vi "QuickSortinData.vi"(0 "line":u16, 2 "plane":u16, 3 "binning [ms]":dbl format="%.2f", 8 "rawdata":T2, 10 "IMAGE Cluster 4":T1) -> (14 "valid":i32, 16 "invalid":u32, 17 "gap":u32, 19 "IMAGE Cluster":T1)   [LabVIEW 2009]
uses:
  ImageCluster.ctl
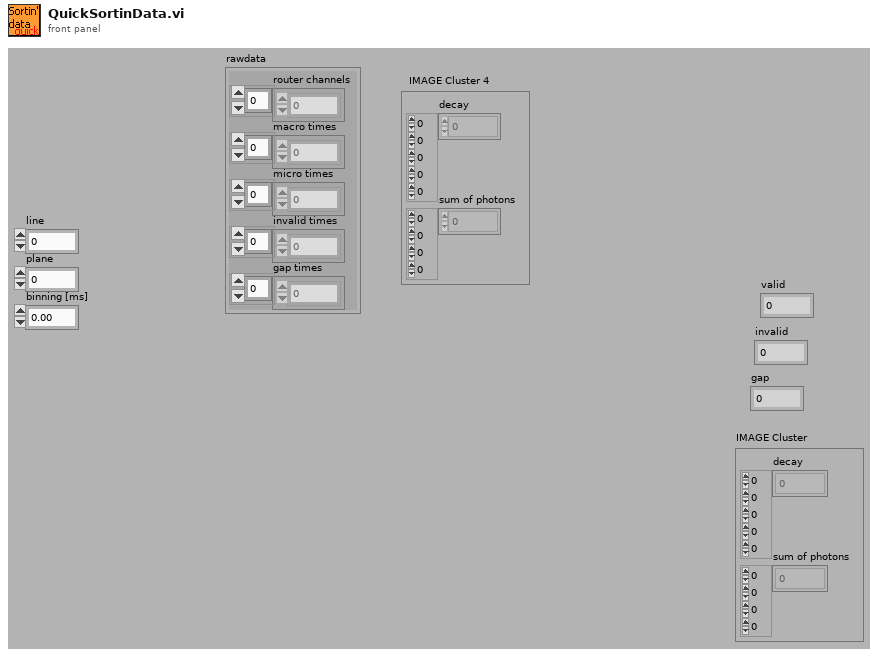
[diagram p1: front panel]
types:
  T1 = typedef "ImageCluster.ctl" = cluster{"decay":u16[][][][][], "sum of photons":u32[][][][]}
  T2 = cluster{"router channels":u8[], "macro times":dbl[], "micro times":u16[], "invalid times":dbl[], "gap times":dbl[]}
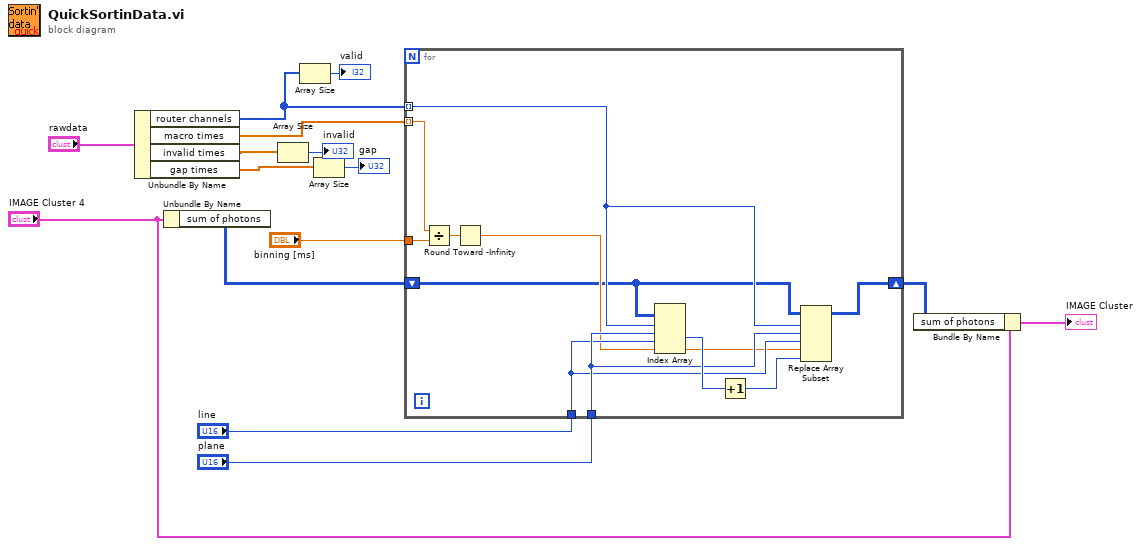
[diagram p0: block diagram]
diagram:
  n1 = Unbundle By Name("rawdata") -> ("router channels"=w5:u8[], "macro times"=w14:dbl[], "invalid times"=w9:dbl[], "gap times"=w8:dbl[])
  n2 = Unbundle By Name("IMAGE Cluster 4") -> ("sum of photons"=w11:u32[][][][])
  n3 = Array Size(array=w9) -> (size(s)=→"invalid":i32)
  n4 = Array Size(array=w5) -> (size(s)=→"valid":i32)
  n5 = Array Size(array=w8) -> (size(s)=→"gap":i32)
  n6 = for {
    tunnel: w5 -> [w23] mode=indexing
    tunnel: w14 -> [w17] mode=indexing
    tunnel: "line" -> [w21]
    tunnel: "plane" -> [w22]
    tunnel: "binning [ms]" -> [w26]
    shift-right: [w18] -> w10
    shift-left: w11 -> [w19]
    n7 = Divide(x=w17, y=w26) -> (x/y=w16:dbl)
    n8 = Round Toward -Infinity(1:w16) -> (0:w20:dbl)
    n9 = Index Array(array=w19, index (dim 0)=w23, index (dim 1)=w22, index (dim 2)=w21, index (dim 3)=w20) -> (element=w25:u32)
    n10 = Increment(x=w25) -> (x+1=w24:u32)
    n11 = Replace Array Subset(array=w19, new element=w24, index (dim 0)=w23, index (dim 1)=w22, index (dim 2)=w21, index (dim 3)=w20) -> (w18:u32[][][][])
  }
  n12 = Bundle By Name(cluster="IMAGE Cluster 4", "sum of photons"=w10) -> (→"IMAGE Cluster":T1)
